vi "Digital Read.vi"(8 "Error In":errorcluster, 10 "DIO Channels":u8[](array[numeric]), 11 "LINX Device Config":T1) -> (0 "Error Out":errorcluster, 2 "Values":bool[](array[boolean]), 3 "LINX Device Config":T1)   [LabVIEW 2011, in "LVH-LINX.lvlib" / "Device.lvlib"]
uses:
  Device.lvlib
  Type Defs/LINX Device Config.ctl
  Type Defs/Interface.ctl
  Type Defs/TCP Config.ctl
  Type Defs/Device Family.ctl
  Type Defs/Error Type.ctl
  LVH-LINX.lvlib
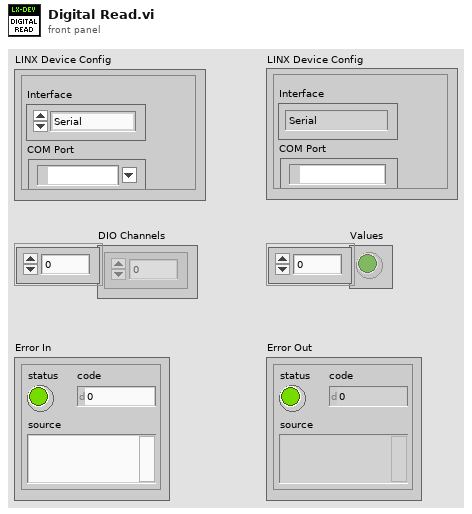
[diagram p1: front panel]
types:
  T1 = typedef "LVH-LINX.lvlib/Device.lvlib/LINX Device Config.ctl" = cluster{"Interface":T2, "COM Port":refnum<visa-resource-name>, "TCP Configuration":T3, "Device Family":T4, "Device ID":u8, "Device Name":string, "TCP Ref":refnum<k5>}
  T2 = typedef "LVH-LINX.lvlib/Interface.ctl" = enum16{"Serial", "TCP"}
  T3 = typedef "LVH-LINX.lvlib/Device.lvlib/TCP Config.ctl" = cluster{"IP Address":string, "Port":u16}
  T4 = typedef "LVH-LINX.lvlib/Device Family.ctl" = enum8{"National Instruments", "Digilent", "Arduino"}
  T5 = typedef "LVH-LINX.lvlib/Error Type.ctl" = enum16{"Unknown", "Timeout", "Corrupt Return Packet", "Unable To Connect", "Command Not Supported", "Channel DNE"}
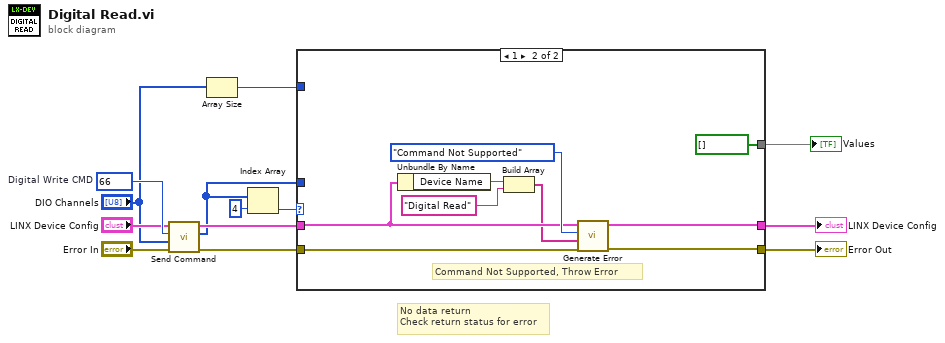
[diagram p0: block diagram]
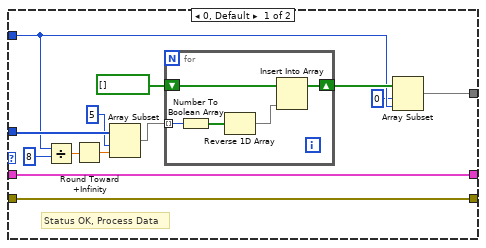
[diagram p2: hidden frame]
diagram:
  w12 = u16 66  # Digital Write CMD
  # "No data return\nCheck return status for error"
  n1 = call "Send Command.vi"("Error In"="Error In", "ARGS"="DIO Channels", "CMD"=w12, "LINX Device Config"="LINX Device Config") -> ("Error Out"=w5:errorcluster, "Response"=w4:u8[], "LINX Device Config"=w7:T1)  [unwired: 5 in]
  n2 = Array Size(array="DIO Channels") -> (size(s)=w2:i32)
  n3 = Index Array(array=w4, index=4) -> (element=w9:u8)
  n4 = case shown="1" w9 {
    tunnel: [w26 w38] -> w8
    tunnel: w7 -> [w26 w33]
    tunnel: [w25 w39] -> w6
    tunnel: w5 -> [w25 w40]
    tunnel: w4 -> [w24 _]
    tunnel: w2 -> [w16 _]
    tunnel: [w14 bool[] []] -> w1
    frame 0, Default {
      # "Status OK, Process Data"
      n5 = Divide(x=w16, y=8) -> (x/y=w22:dbl)
      n6 = Round Toward +Infinity(x=w22) -> (ceil(x): smallest int >= x=w21:dbl)
      n7 = Array Subset(array=w24, index=5, length=w21) -> (w19:u8[])
      n8 = for {
        tunnel: w19 -> [w31] mode=indexing
        shift-right: [w29] -> w17
        shift-left: bool[] [] ("Boolean array") -> [w30]
        n9 = Number To Boolean Array(number=w31) -> (Boolean array=w28:bool[])
        n10 = Reverse 1D Array(array=w28) -> (reversed array=w27:bool[])
        n11 = Insert Into Array(array=w30, new element=w27) -> (w29:bool[])  [unwired: 1 in]
      }
      n12 = Array Subset(array=w17, index=0, length=w16) -> (w14:bool[])
    }
    frame 1 {
      # "Command Not Supported, Throw Error"
      n13 = Unbundle By Name(w33) -> ("Device Name"=w35:string)
      n14 = Build Array(w35, "Digital Read") -> (w32:string[])
      n15 = call "Generate Error.vi"("Error In"=w40, "Arguments"=w32, "Error Type"=Error_Type."Command Not Supported", "LINX Device Config"=w33) -> ("Error Out"=w39:errorcluster, "LINX Device Config"=w38:T1)  [unwired: 6 in]
    }
  }
  "Error Out" <- w6
  "LINX Device Config" <- w8
  "Values" <- w1
